vi "practice2.vi"() -> ()   [LabVIEW 2014]
doc: "This VI demonstrates the individual configuration of settings in I/W, W/I, and continuous operation modes.\n\nThis VI is not meant to be used with infusion-only models. \n\nNotes:\n(1) If continuous mode is selected, infuse volumes/rates will be used."
uses:
  <vilib>/Motion/FlexMotion/CustomControls/CustomControls.llb/AxisOrVectorSpace To Configure.flx
  <vilib>/Motion/FlexMotion/FunctionsVIs/StartStopMotion.llb/Start Motion (8 axes).flx
  <vilib>/Motion/FlexMotion/FunctionsVIs/Trajectory.llb/Check Move Complete Status (8 axes).flx
  <vilib>/Motion/FlexMotion/FunctionsVIs/StartStopMotion.llb/Stop Motion (8 axes).flx
  <instrlib>/KD Scientific 2XX Series/KD Scientific 2XX Series.lvlib
  <vilib>/vision/NI_Vision_Development_Module.lvlib
panel:
  in  "stop (F)":bool
  out "Data from Transducer":dynamicdata(graph) caption="Voltage from Transducer V"
  out "Voltage from pressure transducer":dbl[](array[numeric])
  out "Pressure mm Hg":dbl[](graph)
  in  "Calibration factor":dbl[](array[numeric])
  in  "Zero Error":dbl[](array[numeric])
  out "pressure mm Hg":dbl[](array[numeric])
  in  "stop 2":bool
  out "Voltage (V)":dbl=0.3869919147841388
  out "Force (grams)":dbl=0.3869919147841388
  out "Force Graph (g)":dynamicdata(graph)
  in  "Zero":dbl=-99.6 format="%#_13g"
  out "Load Cell Output (mV)":dynamicdata(graph)
  in  "Displacement in mm":dbl
  in  "Velocity in mm/s":dbl
  out "Image":T1(plugin-control)
  out "Particle Measurements (Pixels) (Particle Analysis 1)":dbl[][](array[numeric]) format="%.2f"
  out "subarray":dbl[](array[numeric])
  out "The diameter":dbl[](array[numeric])
  out "Image from  Vision Acquisition 1":T1(plugin-control)
  out "Units":string
  out "Delivered Volume":dbl
  in  "stop":bool
  out "Status":T2
  in  "Baud Rate (9600)":u32(ring)=9600 items=["300"=300, "1200"=1200, "2400"=2400, "4800"=4800, "9600"=9600]
  in  "Withdrawal Settings":T3={"Flow Rate (5)"=5.0, "Volume (10)"=10.0, "Volume Units (ml)"=enum."milliliters (ml)", "Rate Units (ml/min.)"=enum."milliliters per minute (ml/min.)"} {"Volume (10)" format="%#.3g"}
  in  "Diameter (8.75 mm)":dbl=8.75
  in  "Infusion Settings":T3={"Flow Rate (5)"=5.0, "Volume (10)"=10.0, "Volume Units (ml)"=enum."milliliters (ml)", "Rate Units (ml/min.)"=enum."milliliters per minute (ml/min.)"}
  in  "Operation Mode (Infuse)":u16(ring) items=["Infuse", "Withdraw", "Infuse-Withdraw", "Withdraw-Infuse", "Continuous"]
  in  "Address (0)":i32 format="%0.0f"
  in  "error in (no error)":errorcluster
  in  "VISA resource name":refnum<visa-resource-name>="COM1"
  # "CCD Camera Input"
  # "Load Cell Input"
  # "Syringe Pump Control"
  # "RS-232 Settings"
  # "General Settings"
  # "Pump Status"
  # "Displacement Motor Control"
  # "Pressure Transducer"
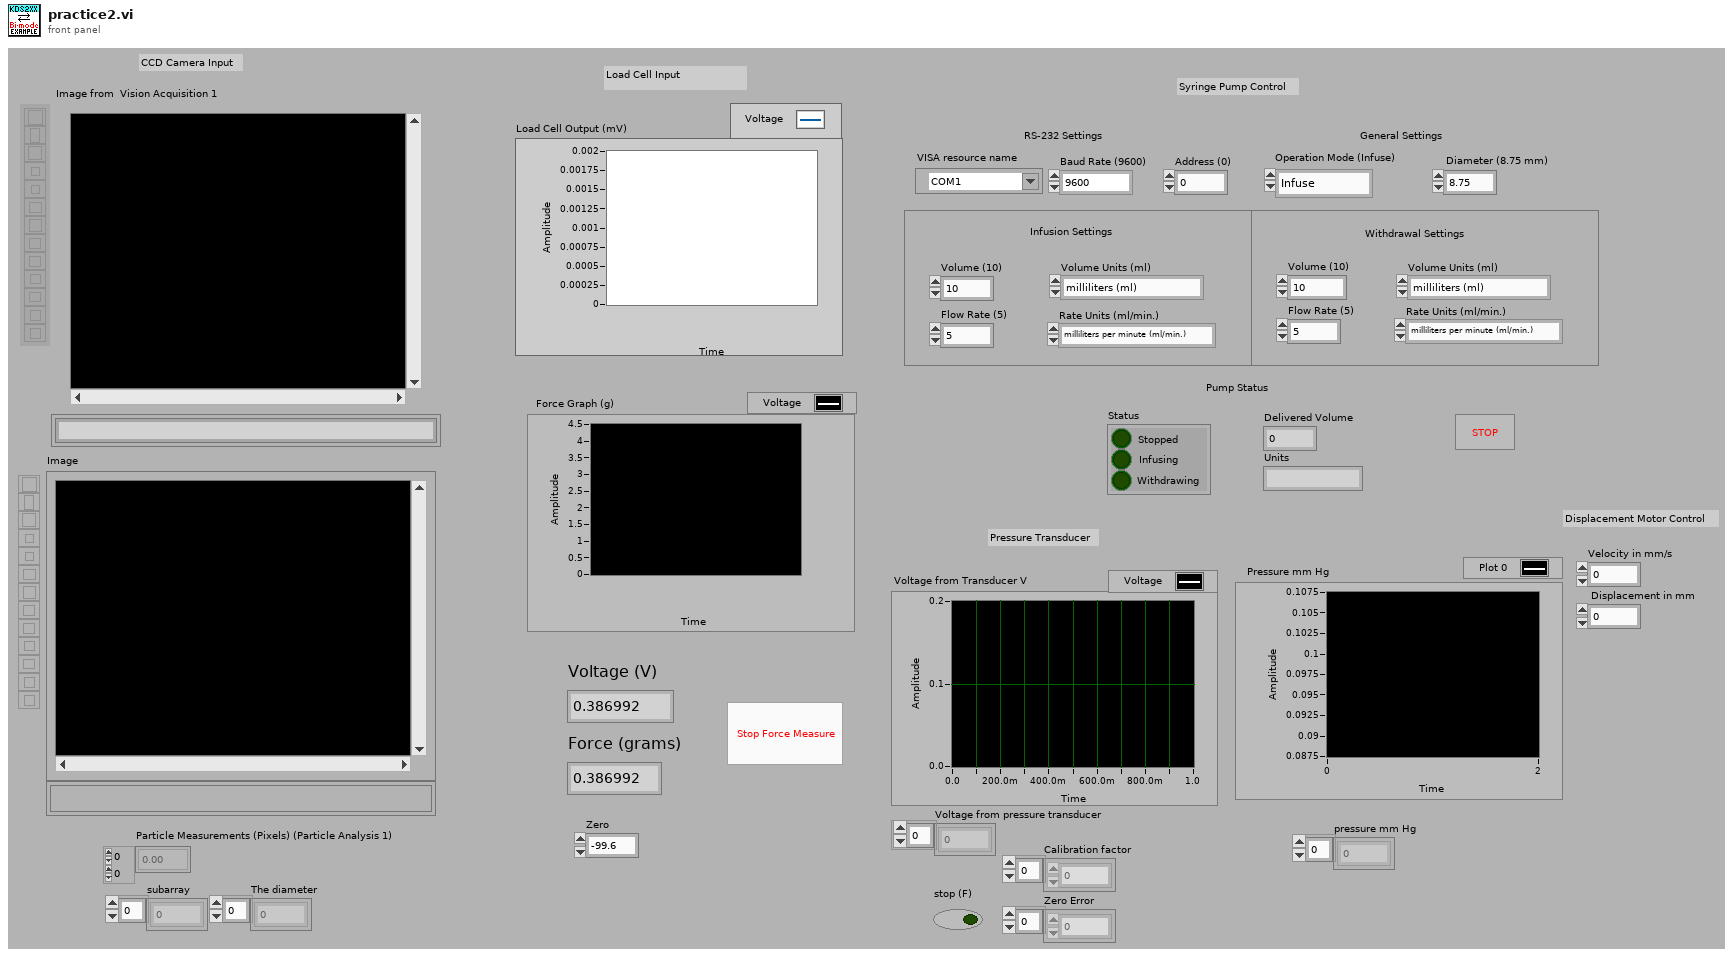
[diagram p1: front panel]
types:
  T1 = typedef "IMAQ Image.ctl" = refnum<image>
  T2 = cluster{"Stopped":bool, "Infusing":bool, "Withdrawing":bool}
  T3 = cluster{"Flow Rate (5)":dbl, "Volume (10)":dbl, "Volume Units (ml)":enum16{"milliliters (ml)", "microliters (ul)"}, "Rate Units (ml/min.)":enum16{"milliliters per minute (ml/min.)", "milliliters per hour (ml/hr.)", "microliters per minute (ul/min.)", "microliters per hour (ul/hr.)"}}
  T4 = typedef "Board Id" = u8
  T5 = enum16{"Absolute Position", "Relative Position", "Velocity", "Relative to Cap Pos", "Modulus Position", "Absolute Contouring", "Relative Contouring"}
  T6 = typedef "ROI Descriptor" = cluster{"Global Rectangle":i32[], "Contours":cluster{"ID":enum32{"External", "Internal"}, "Type":u32, "Coordinates":i32[]}[]}
  T7 = typedef "AxisOrVectorSpace To Configure.flx" = u16
  T8 = typedef "Resource Out (Enum).flx" = u16
  T9 = typedef "Bd Id Out" = u8
  T10 = enum16{"milliliters per minute (ml/min.)", "milliliters per hour (ml/hr.)", "microliters per minute (ul/min.)", "microliters per hour (ul/hr.)"}
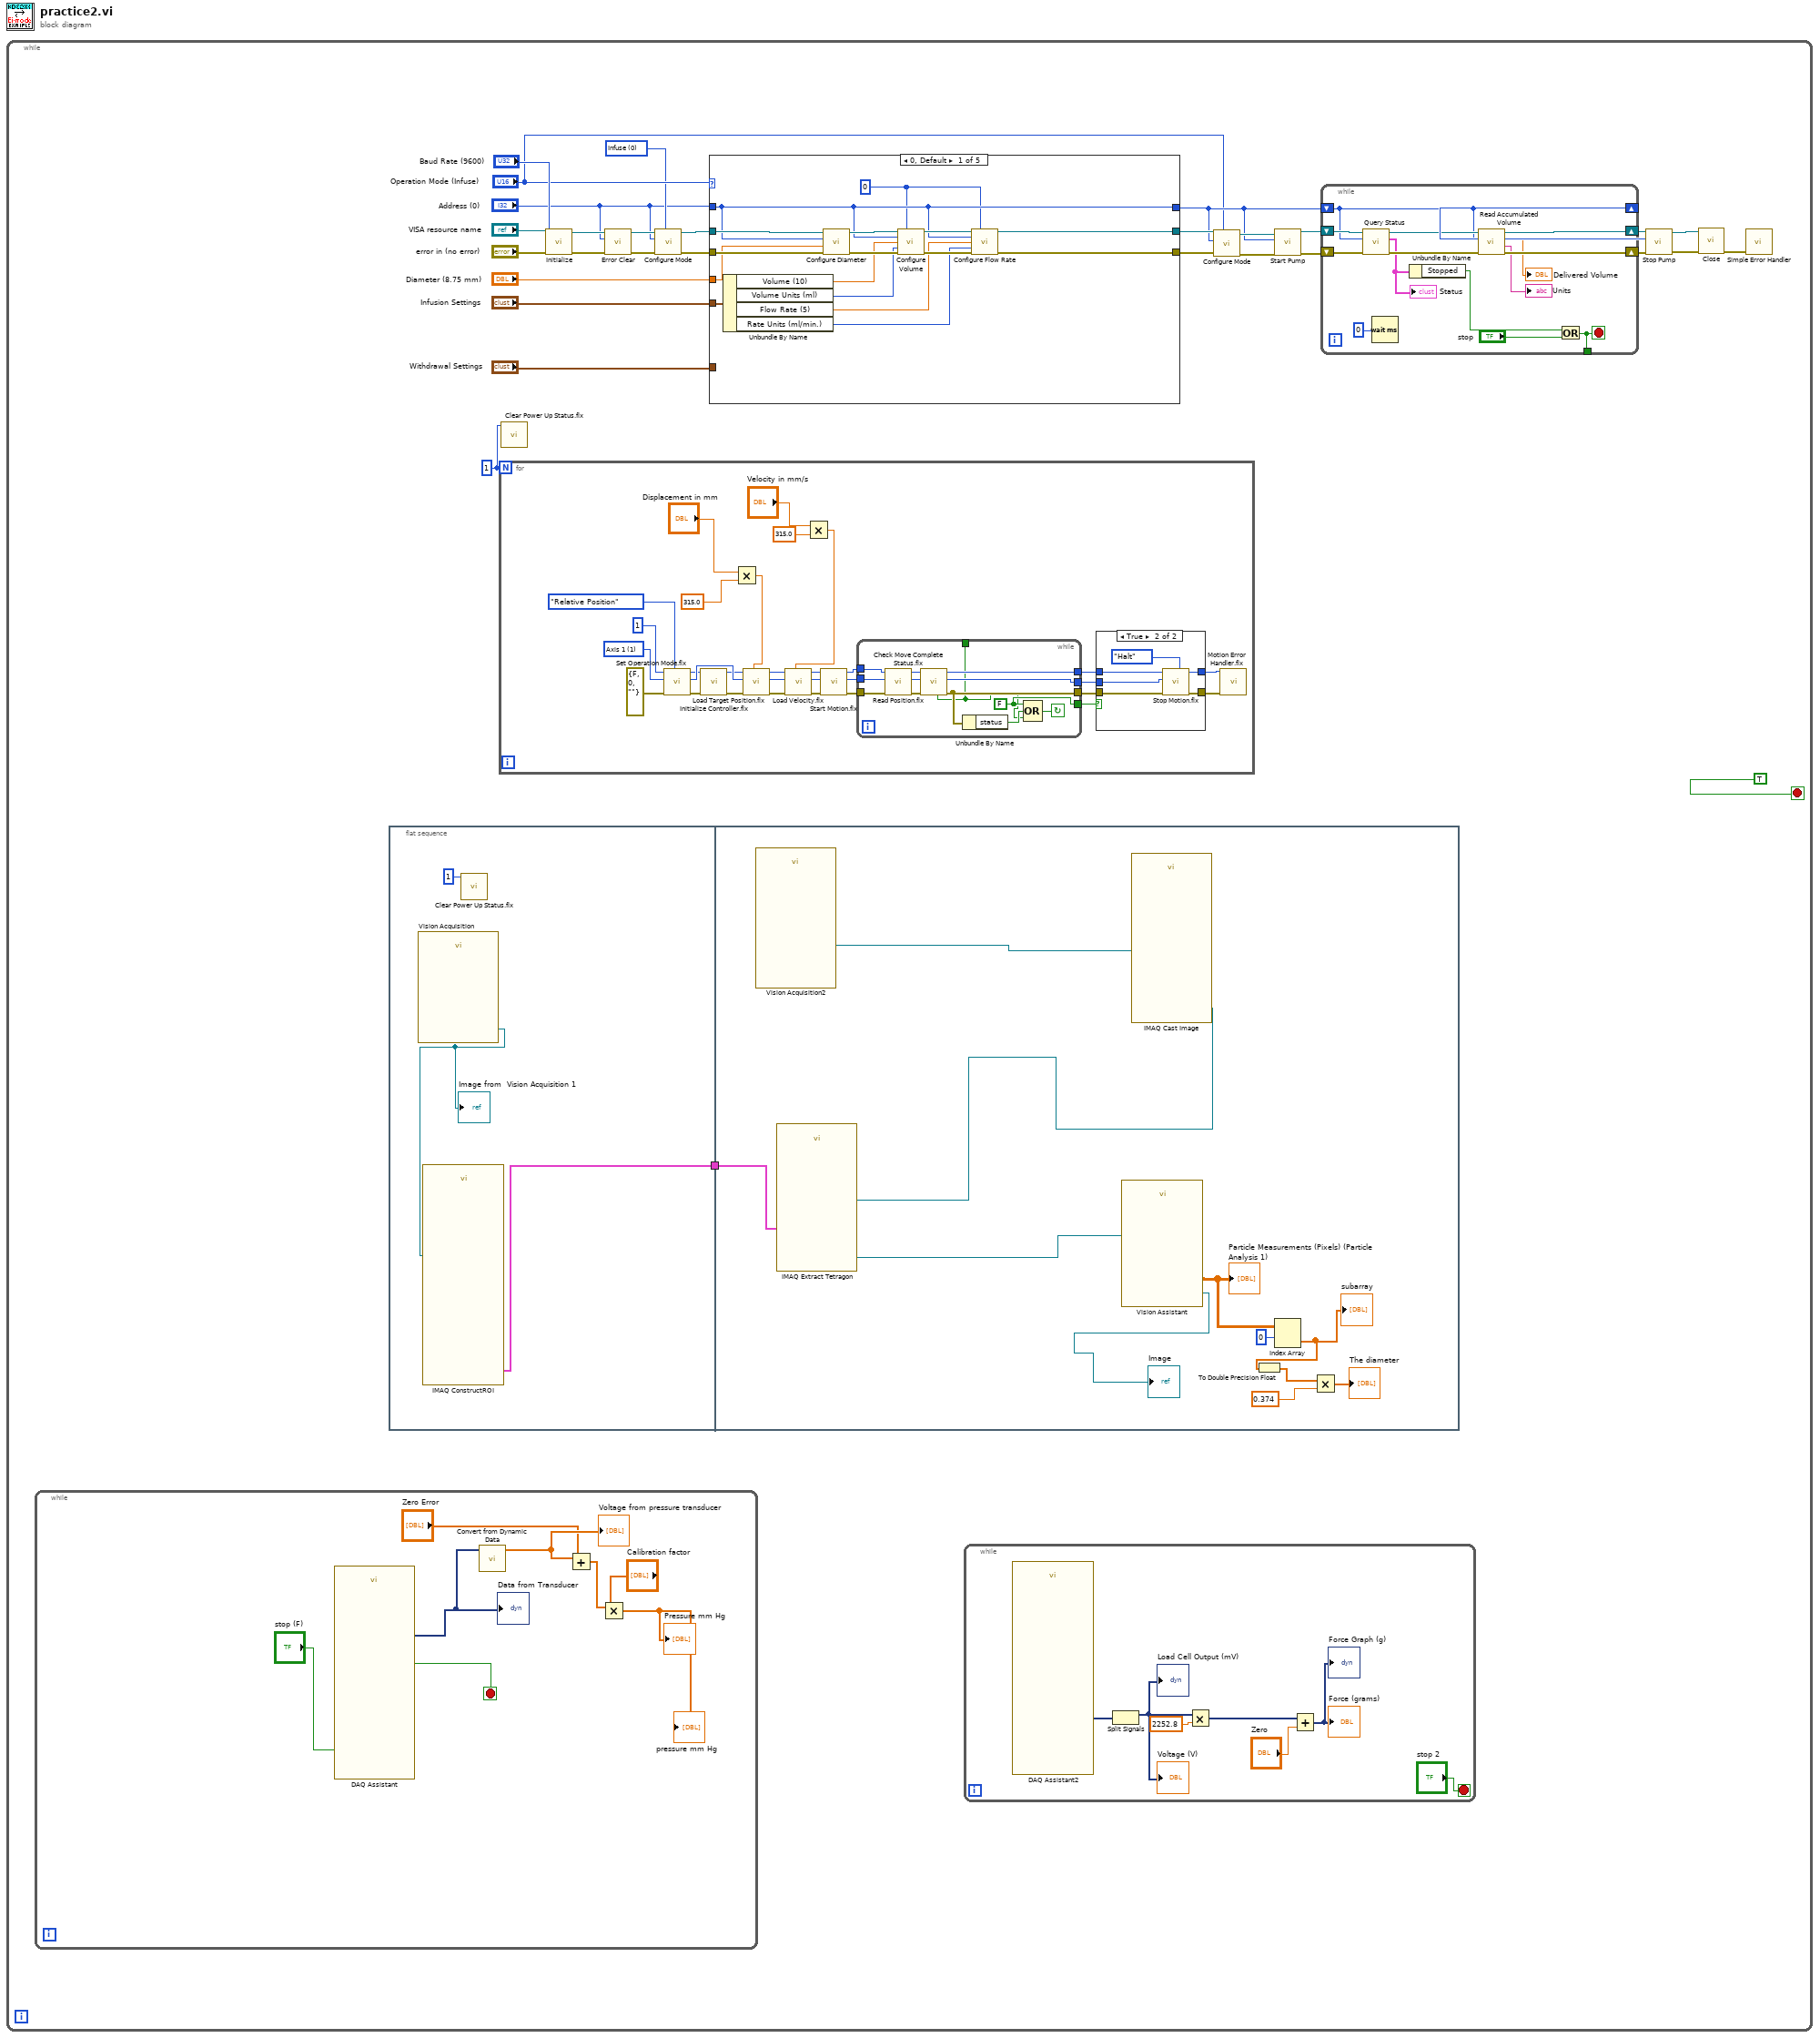
[diagram p0: block diagram]
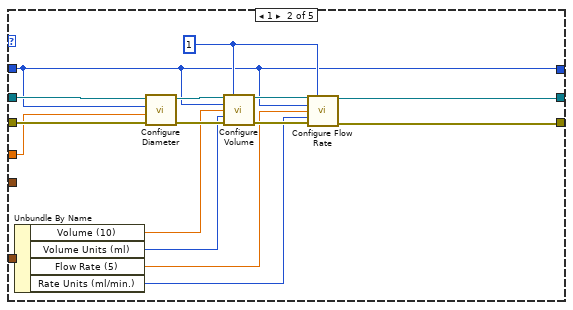
[diagram p3: hidden frame]
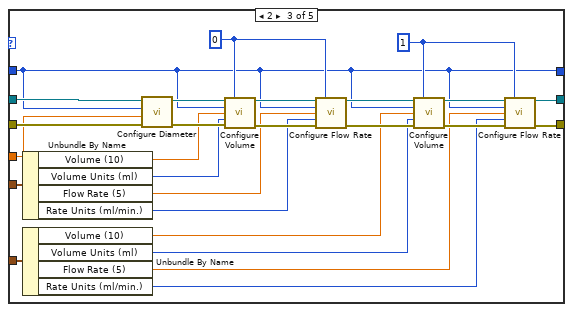
[diagram p4: hidden frame]
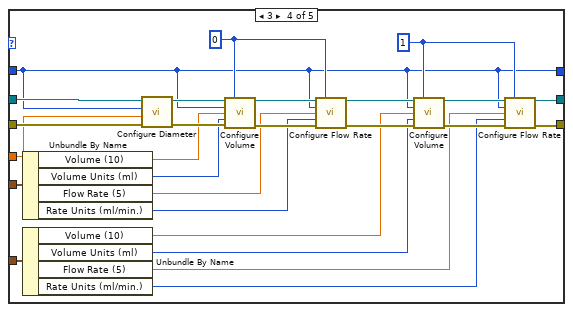
[diagram p5: hidden frame]
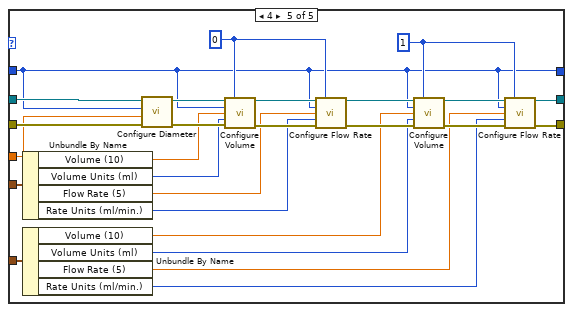
[diagram p6: hidden frame]
diagram:
  n1 = while {
    stop <- TRUE stop-if-true
    w3 = T4 1 ("Board ID")
    w9 = u16 0 items=["Infuse", "Withdraw", "Infuse-Withdraw", "Withdraw-Infuse", "Continuous"] ("Mode (infuse)")
    n2 = flat-sequence {
      tunnel: [w41] -> w1
      tunnel: w1 -> [w52]
      frame #0 {
        n3 = call "Vision Acquisition"() -> ("Image Out"=w39:T1)  [unwired: 26 in, 1 out]
        "Image from  Vision Acquisition 1" <- w39
        n4 = call "IMAQ ConstructROI"("Image"=w39) -> ("ROI Descriptor Out"=w41:T6)  [unwired: 7 in, 3 out]
        n5 = call <vilib>:"Clear Power Up Status.flx"("Board ID"=T4 1) -> ()  [unwired: 6 in, 2 out]
      }
      frame #1 {
        n6 = call "Vision Acquisition2"() -> ("Image Out"=w50:T1)  [unwired: 25 in, 2 out]
        n7 = call "IMAQ Cast Image"("Image Src"=w50) -> ("Image Dst Out"=w48:T1)  [unwired: 9 in, 1 out]
        n8 = call-poly "IMAQ Extract Tetragon"("ROI Descriptor"=w52, "Image Src"=w48) -> ("Image Dst Out"=w49:T1)  [unwired: 8 in, 1 out]
        n9 = call "Vision Assistant"("Image In"=w49) -> ("Image Out"=→"Image":T1, "Particle Measurements (Pixels) (Particle Analysis 1)"=w47:dbl[][])  [unwired: 23 in, 2 out]
        "Particle Measurements (Pixels) (Particle Analysis 1)" <- w47
        n10 = Index Array(array=w47, index (row)=0) -> (element=w45:dbl[])  [unwired: 1 in]
        "subarray" <- w45
        n11 = To Double Precision Float(number=w45) -> (double precision float=w44:dbl[])
        n12 = Multiply(x=w44, y=0.374) -> (x*y=→"The diameter":dbl[])
      }
    }
    n13 = for {
      N: w3 -> [_]
      w80 = T7 1 items=["Axis 1"=1, "Axis 2"=2, "Axis 3"=3, "Axis 4"=4, "Axis 5"=5, "Axis 6"=6, "Axis 7"=7, "Axis 8"=8, "Vector Space 1"=17, "Vector Space 2"=18, "Vector Space 3"=19, "Vector Space 4"=20] ("Axis or Vector Space")
      n14 = call <vilib>:"Set Operation Mode.flx"("Position Mode (Absolute)"=T5."Relative Position", "error in (no error)"=errorcluster {"status"=FALSE, "code"=0, "source"=""} ("error constant"), "Axis or Vector Space"=w80, "Board ID"=T4 1) -> ("error out"=w78:errorcluster, "Resource Output"=w77:T8, "Bd ID Out"=w76:T9)  [unwired: 2 in]
      n15 = call <vilib>:"Initialize Controller.flx"("error in (no error)"=w78, "Board ID"=w76) -> ("error out"=w71:errorcluster, "Bd ID Out"=w75:T9)  [unwired: 6 in]
      n16 = Multiply(x="Displacement in mm", y=315.0) -> (x*y=w55:dbl)
      n17 = call <vilib>:"Load Target Position.flx"("Target Position (0)"=w55, "error in (no error)"=w71, "Axis"=w77, "Board ID"=w75) -> ("error out"=w72:errorcluster, "Resource Output"=w73:T8, "Bd ID Out"=w74:T9)  [unwired: 3 in]
      n18 = Multiply(x="Velocity in mm/s", y=315.0) -> (x*y=w56:dbl)
      n19 = call <vilib>:"Load Velocity.flx"("Velocity (10000)"=w56, "error in (no error)"=w72, "Axis or Vector Space"=w73, "Board ID"=w74) -> ("error out"=w68:errorcluster, "Resource Output"=w69:T8, "Bd ID Out"=w70:T9)  [unwired: 3 in]
      n20 = call-poly <vilib>:"Start Motion.flx"("error in (no error)"=w68, "Axis or Vector Space"=w69, "Board ID"=w70) -> ("error out"=w65:errorcluster, "Resource Output"=w66:T8, "Bd ID Out"=w67:T9)  [unwired: 3 in]
      n21 = while {
        tunnel: w67 -> [w103]
        tunnel: w66 -> [w102]
        tunnel: w65 -> [w101]
        tunnel: [w96] -> w64
        tunnel: [w95] -> w63
        tunnel: [w93] -> w62
        tunnel: [w92] -> w61
        tunnel: [w91] -> _
        stop <- w97 continue-if-true
        w96 = FALSE
        n22 = call <vilib>:"Read Position.flx"("error in (no error)"=w101, "Axis"=w102, "Board ID"=w103) -> ("error out"=w98:errorcluster, "Resource Output"=w99:T8, "Bd ID Out"=w100:T9)  [unwired: 3 in, 1 out]
        n23 = call-poly <vilib>:"Check Move Complete Status.flx"("error in (no error)"=w98, "Axis or Vector Space"=w99, "Board ID"=w100) -> ("error out"=w95:errorcluster, "Resource Output"=w92:T8, "Bd ID Out"=w93:T9, "Move Complete"=w91:bool)  [unwired: 3 in]
        n24 = Unbundle By Name(w95) -> ("status"=w94:bool)
        n25 = Compound Arithmetic op=OR(w96, w94, w91) -> (w97:bool)
      }
      n26 = case shown="True" w64 {
        tunnel: w63 -> [w83 w89]
        tunnel: w62 -> [w84 w88]
        tunnel: w61 -> [_ w87]
        tunnel: [w83 w86] -> w60
        tunnel: [w84 w85] -> w59
        frame False {
        }
        frame True {
          n27 = call-poly <vilib>:"Stop Motion.flx"("Stop Type (Decel)"=enum16{"Decelerate", "Halt", "Kill"}."Halt", "error in (no error)"=w89, "Axis or Vector Space"=w87, "Board ID"=w88) -> ("error out"=w86:errorcluster, "Bd ID Out"=w85:T9)  [unwired: 3 in, 1 out]
        }
      }
      n28 = call <vilib>:"Motion Error Handler.flx"("Board ID"=w59, "error in (no error)"=w60) -> ()  [unwired: 9 in, 5 out]
    }
    n29 = call <vilib>:"Clear Power Up Status.flx"("Board ID"=w3) -> ()  [unwired: 6 in, 2 out]
    n30 = call <instrlib>:"Initialize.vi"("error in (no error)"="error in (no error)", "Baud Rate (9600)"="Baud Rate (9600)", "VISA resource name"="VISA resource name") -> ("error out"=w6:errorcluster, "VISA resource name out"=w5:refnum<visa-resource-name>)  [unwired: 7 in]
    n31 = call <instrlib>:"Error Clear.vi"("error in (no error)"=w6, "Address (0)"="Address (0)", "VISA resource name"=w5) -> ("error out"=w7:errorcluster, "VISA resource name out"=w8:refnum<visa-resource-name>)  [unwired: 6 in, 1 out]
    n32 = call <instrlib>:"Configure Mode.vi"("Mode (infuse)"=w9, "error in (no error)"=w7, "Address (0)"="Address (0)", "VISA resource name"=w8) -> ("error out"=w11:errorcluster, "VISA resource name out"=w10:refnum<visa-resource-name>)  [unwired: 6 in]
    n33 = case shown="0, Default" "Operation Mode (Infuse)" {
      tunnel: "Infusion Settings" -> [w113 _ w161 w187 w213]
      tunnel: "Withdrawal Settings" -> [_ w135 w160 w186 w212]
      tunnel: w10 -> [w119 w134 w159 w185 w211]
      tunnel: w11 -> [w118 w130 w158 w184 w210]
      tunnel: "Diameter (8.75 mm)" -> [w112 w126 w141 w167 w193]
      tunnel: [w111 w120 w136 w162 w188] -> w13
      tunnel: "Address (0)" -> [w111 w120 w136 w162 w188]
      tunnel: [w106 w131 w138 w164 w190] -> w17
      tunnel: [w105 w127 w137 w163 w189] -> w16
      frame 0, Default {
        w104 = 0
        n34 = Unbundle By Name(w113) -> ("Volume (10)"=w110:dbl, "Volume Units (ml)"=w109:enum16{"milliliters (ml)", "microliters (ul)"}, "Flow Rate (5)"=w108:dbl, "Rate Units (ml/min.)"=w107:T10)
        n35 = call <instrlib>:"Configure Diameter.vi"("error in (no error)"=w118, "Diameter (8.75 mm)"=w112, "Address (0)"=w111, "VISA resource name"=w119) -> ("error out"=w116:errorcluster, "VISA resource name out"=w117:refnum<visa-resource-name>)  [unwired: 6 in]
        n36 = call <instrlib>:"Configure Volume.vi"("VISA resource name"=w117, "Mode (infuse)"=w104, "Address (0)"=w111, "Volume (100)"=w110, "Units (0: milliliters)"=w109, "error in (no error)"=w116) -> ("VISA resource name out"=w115:refnum<visa-resource-name>, "error out"=w114:errorcluster)  [unwired: 8 in]
        n37 = call <instrlib>:"Configure Flow Rate.vi"("VISA resource name"=w115, "Mode (infuse)"=w104, "Address (0)"=w111, "Flow Rate (5)"=w108, "Units (0: milliliters per minute)"=w107, "error in (no error)"=w114) -> ("VISA resource name out"=w106:refnum<visa-resource-name>, "error out"=w105:errorcluster)  [unwired: 8 in]
      }
      frame 1 {
        w121 = 1
        n38 = Unbundle By Name(w135) -> ("Volume (10)"=w125:dbl, "Volume Units (ml)"=w124:enum16{"milliliters (ml)", "microliters (ul)"}, "Flow Rate (5)"=w123:dbl, "Rate Units (ml/min.)"=w122:T10)
        n39 = call <instrlib>:"Configure Diameter.vi"("error in (no error)"=w130, "Diameter (8.75 mm)"=w126, "Address (0)"=w120, "VISA resource name"=w134) -> ("error out"=w129:errorcluster, "VISA resource name out"=w133:refnum<visa-resource-name>)  [unwired: 6 in]
        n40 = call <instrlib>:"Configure Volume.vi"("VISA resource name"=w133, "Mode (infuse)"=w121, "Address (0)"=w120, "Volume (100)"=w125, "Units (0: milliliters)"=w124, "error in (no error)"=w129) -> ("VISA resource name out"=w132:refnum<visa-resource-name>, "error out"=w128:errorcluster)  [unwired: 8 in]
        n41 = call <instrlib>:"Configure Flow Rate.vi"("VISA resource name"=w132, "Mode (infuse)"=w121, "Address (0)"=w120, "Flow Rate (5)"=w123, "Units (0: milliliters per minute)"=w122, "error in (no error)"=w128) -> ("VISA resource name out"=w131:refnum<visa-resource-name>, "error out"=w127:errorcluster)  [unwired: 8 in]
      }
      frame 2 {
        w139 = 1
        w140 = 0
        n42 = Unbundle By Name(w161) -> ("Volume (10)"=w149:dbl, "Volume Units (ml)"=w148:enum16{"milliliters (ml)", "microliters (ul)"}, "Flow Rate (5)"=w147:dbl, "Rate Units (ml/min.)"=w146:T10)
        n43 = Unbundle By Name(w160) -> ("Volume (10)"=w145:dbl, "Volume Units (ml)"=w144:enum16{"milliliters (ml)", "microliters (ul)"}, "Flow Rate (5)"=w143:dbl, "Rate Units (ml/min.)"=w142:T10)
        n44 = call <instrlib>:"Configure Diameter.vi"("error in (no error)"=w158, "Diameter (8.75 mm)"=w141, "Address (0)"=w136, "VISA resource name"=w159) -> ("error out"=w153:errorcluster, "VISA resource name out"=w157:refnum<visa-resource-name>)  [unwired: 6 in]
        n45 = call <instrlib>:"Configure Volume.vi"("VISA resource name"=w157, "Mode (infuse)"=w140, "Address (0)"=w136, "Volume (100)"=w149, "Units (0: milliliters)"=w148, "error in (no error)"=w153) -> ("VISA resource name out"=w156:refnum<visa-resource-name>, "error out"=w152:errorcluster)  [unwired: 8 in]
        n46 = call <instrlib>:"Configure Flow Rate.vi"("VISA resource name"=w156, "Mode (infuse)"=w140, "Address (0)"=w136, "Flow Rate (5)"=w147, "Units (0: milliliters per minute)"=w146, "error in (no error)"=w152) -> ("VISA resource name out"=w155:refnum<visa-resource-name>, "error out"=w151:errorcluster)  [unwired: 8 in]
        n47 = call <instrlib>:"Configure Volume.vi"("VISA resource name"=w155, "Mode (infuse)"=w139, "Address (0)"=w136, "Volume (100)"=w145, "Units (0: milliliters)"=w144, "error in (no error)"=w151) -> ("VISA resource name out"=w154:refnum<visa-resource-name>, "error out"=w150:errorcluster)  [unwired: 8 in]
        n48 = call <instrlib>:"Configure Flow Rate.vi"("VISA resource name"=w154, "Mode (infuse)"=w139, "Address (0)"=w136, "Flow Rate (5)"=w143, "Units (0: milliliters per minute)"=w142, "error in (no error)"=w150) -> ("VISA resource name out"=w138:refnum<visa-resource-name>, "error out"=w137:errorcluster)  [unwired: 8 in]
      }
      frame 3 {
        w165 = 1
        w166 = 0
        n49 = Unbundle By Name(w187) -> ("Volume (10)"=w175:dbl, "Volume Units (ml)"=w174:enum16{"milliliters (ml)", "microliters (ul)"}, "Flow Rate (5)"=w173:dbl, "Rate Units (ml/min.)"=w172:T10)
        n50 = Unbundle By Name(w186) -> ("Volume (10)"=w171:dbl, "Volume Units (ml)"=w170:enum16{"milliliters (ml)", "microliters (ul)"}, "Flow Rate (5)"=w169:dbl, "Rate Units (ml/min.)"=w168:T10)
        n51 = call <instrlib>:"Configure Diameter.vi"("error in (no error)"=w184, "Diameter (8.75 mm)"=w167, "Address (0)"=w162, "VISA resource name"=w185) -> ("error out"=w179:errorcluster, "VISA resource name out"=w183:refnum<visa-resource-name>)  [unwired: 6 in]
        n52 = call <instrlib>:"Configure Volume.vi"("VISA resource name"=w183, "Mode (infuse)"=w166, "Address (0)"=w162, "Volume (100)"=w175, "Units (0: milliliters)"=w174, "error in (no error)"=w179) -> ("VISA resource name out"=w182:refnum<visa-resource-name>, "error out"=w178:errorcluster)  [unwired: 8 in]
        n53 = call <instrlib>:"Configure Flow Rate.vi"("VISA resource name"=w182, "Mode (infuse)"=w166, "Address (0)"=w162, "Flow Rate (5)"=w173, "Units (0: milliliters per minute)"=w172, "error in (no error)"=w178) -> ("VISA resource name out"=w181:refnum<visa-resource-name>, "error out"=w177:errorcluster)  [unwired: 8 in]
        n54 = call <instrlib>:"Configure Volume.vi"("VISA resource name"=w181, "Mode (infuse)"=w165, "Address (0)"=w162, "Volume (100)"=w171, "Units (0: milliliters)"=w170, "error in (no error)"=w177) -> ("VISA resource name out"=w180:refnum<visa-resource-name>, "error out"=w176:errorcluster)  [unwired: 8 in]
        n55 = call <instrlib>:"Configure Flow Rate.vi"("VISA resource name"=w180, "Mode (infuse)"=w165, "Address (0)"=w162, "Flow Rate (5)"=w169, "Units (0: milliliters per minute)"=w168, "error in (no error)"=w176) -> ("VISA resource name out"=w164:refnum<visa-resource-name>, "error out"=w163:errorcluster)  [unwired: 8 in]
      }
      frame 4 {
        w191 = 1
        w192 = 0
        n56 = Unbundle By Name(w213) -> ("Volume (10)"=w201:dbl, "Volume Units (ml)"=w200:enum16{"milliliters (ml)", "microliters (ul)"}, "Flow Rate (5)"=w199:dbl, "Rate Units (ml/min.)"=w198:T10)
        n57 = Unbundle By Name(w212) -> ("Volume (10)"=w197:dbl, "Volume Units (ml)"=w196:enum16{"milliliters (ml)", "microliters (ul)"}, "Flow Rate (5)"=w195:dbl, "Rate Units (ml/min.)"=w194:T10)
        n58 = call <instrlib>:"Configure Diameter.vi"("error in (no error)"=w210, "Diameter (8.75 mm)"=w193, "Address (0)"=w188, "VISA resource name"=w211) -> ("error out"=w205:errorcluster, "VISA resource name out"=w209:refnum<visa-resource-name>)  [unwired: 6 in]
        n59 = call <instrlib>:"Configure Volume.vi"("VISA resource name"=w209, "Mode (infuse)"=w192, "Address (0)"=w188, "Volume (100)"=w201, "Units (0: milliliters)"=w200, "error in (no error)"=w205) -> ("VISA resource name out"=w208:refnum<visa-resource-name>, "error out"=w204:errorcluster)  [unwired: 8 in]
        n60 = call <instrlib>:"Configure Flow Rate.vi"("VISA resource name"=w208, "Mode (infuse)"=w192, "Address (0)"=w188, "Flow Rate (5)"=w199, "Units (0: milliliters per minute)"=w198, "error in (no error)"=w204) -> ("VISA resource name out"=w207:refnum<visa-resource-name>, "error out"=w203:errorcluster)  [unwired: 8 in]
        n61 = call <instrlib>:"Configure Volume.vi"("VISA resource name"=w207, "Mode (infuse)"=w191, "Address (0)"=w188, "Volume (100)"=w197, "Units (0: milliliters)"=w196, "error in (no error)"=w203) -> ("VISA resource name out"=w206:refnum<visa-resource-name>, "error out"=w202:errorcluster)  [unwired: 8 in]
        n62 = call <instrlib>:"Configure Flow Rate.vi"("VISA resource name"=w206, "Mode (infuse)"=w191, "Address (0)"=w188, "Flow Rate (5)"=w195, "Units (0: milliliters per minute)"=w194, "error in (no error)"=w202) -> ("VISA resource name out"=w190:refnum<visa-resource-name>, "error out"=w189:errorcluster)  [unwired: 8 in]
      }
    }
    n63 = while {
      stop <- "stop 2" stop-if-true
      n64 = call "DAQ Assistant2"() -> ("data"=w37:dynamicdata)  [unwired: 16 in, 3 out]
      n65 = Split Signals(w37) -> (w32:dynamicdata)  [unwired: 2 in, 1 out]
      "Voltage (V)" <- w32
      "Load Cell Output (mV)" <- w32
      n66 = Multiply(x=w32, y=2252.8) -> (x*y=w36:dynamicdata)
      n67 = Add(x=w36, y="Zero") -> (x+y=→"Force (grams)" →"Force Graph (g)":dynamicdata)
    }
    n68 = call <instrlib>:"Configure Mode.vi"("Mode (infuse)"="Operation Mode (Infuse)", "error in (no error)"=w16, "Address (0)"=w13, "VISA resource name"=w17) -> ("error out"=w14:errorcluster, "VISA resource name out"=w15:refnum<visa-resource-name>)  [unwired: 6 in]
    n69 = call <instrlib>:"Start Pump.vi"("error in (no error)"=w14, "Address (0)"=w13, "VISA resource name"=w15) -> ("error out"=w28:errorcluster, "VISA resource name out"=w29:refnum<visa-resource-name>)  [unwired: 7 in]
    n70 = while {
      shift-right: [w217] -> w22
      shift-left: w13 -> [w217]
      shift-right: [w219] -> w27
      shift-left: w29 -> [w224]
      shift-right: [w218] -> w26
      shift-left: w28 -> [w225]
      tunnel: [w214] -> _
      stop <- w214 stop-if-true
      n71 = call <instrlib>:"Query Status.vi"("error in (no error)"=w225, "Address (0)"=w217, "VISA resource name"=w224) -> ("error out"=w227:errorcluster, "Status"=w223:T2, "VISA resource name out"=w220:refnum<visa-resource-name>)  [unwired: 6 in]
      "Status" <- w223
      n72 = Wait (ms)(milliseconds to wait=u32 0) -> ()  [unwired: 1 out]
      n73 = Unbundle By Name(w223) -> ("Stopped"=w222:bool)
      n74 = call <instrlib>:"Read Accumulated Volume.vi"("error in (no error)"=w227, "Address (0)"=w217, "VISA resource name"=w220) -> ("error out"=w218:errorcluster, "Units"=→"Units":string, "Delivered Volume"=→"Delivered Volume":dbl, "VISA resource name out"=w219:refnum<visa-resource-name>)  [unwired: 5 in]
      n75 = Or(x=w222, y="stop") -> (x .or. y?=w214:bool)
    }
    n76 = call <instrlib>:"Stop Pump.vi"("error in (no error)"=w26, "Address (0)"=w22, "VISA resource name"=w27) -> ("error out"=w20:errorcluster, "VISA resource name out"=w19:refnum<visa-resource-name>)  [unwired: 7 in]
    n77 = call <instrlib>:"Close.vi"("error in (no error)"=w20, "VISA resource name"=w19) -> ("error out"=w21:errorcluster)  [unwired: 9 in]
    n78 = call <vilib>:"Simple Error Handler.vi"("error in (no error)"=w21) -> ()  [unwired: 4 in, 5 out]
  }
  n79 = while {
    stop <- w234 stop-if-true
    n80 = call "DAQ Assistant"("stop (F)"="stop (F)") -> ("data"=w233:dynamicdata, "stopped"=w234:bool)  [unwired: 15 in, 2 out]
    "Data from Transducer" <- w233
    n81 = call "Convert from Dynamic Data"("Dynamic Data Type"=w233) -> ("Array"=w230:dbl[])  [unwired: 3 in]
    "Voltage from pressure transducer" <- w230
    n82 = Add(x=w230, y="Zero Error") -> (x+y=w228:dbl[])
    n83 = Multiply(x=w228, y="Calibration factor") -> (x*y=→"Pressure mm Hg" →"pressure mm Hg":dbl[])
  }
